vi "dfd_Normalization.vi"(1 "scale type":T1, 2 "h(n)":dbl[](array[numeric])) -> (0 "norm":dbl)   [LabVIEW 2017, in "NI_DigFilterLicensed.lvlib"]
uses:
  <vilib>/addons/Digital Filter Design/NI_DigFilterLicensed.lvlib
  <vilib>/addons/Digital Filter Design/_Objects.llb/DFD Coef Norm Type.ctl
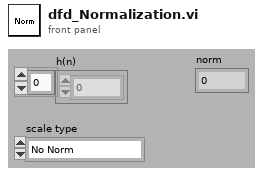
[diagram p1: front panel]
types:
  T1 = typedef "NI_DigFilterLicensed.lvlib/DFD Coef Norm Type.ctl" = enum16{"No Norm", "Time Domain 1-Norm", "Time Domain 2-Norm", "Time Domain Inf-Norm"}
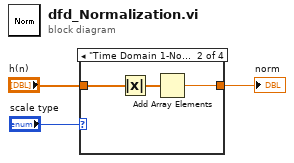
[diagram p0: block diagram]
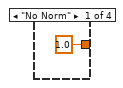
[diagram p2: hidden frame]
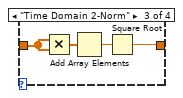
[diagram p3: hidden frame]
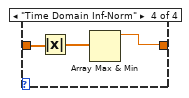
[diagram p4: hidden frame]
diagram:
  n1 = case shown="\"Time Domain 1-Norm\", Default" "scale type" {
    tunnel: "h(n)" -> [_ w7 w11 w14]
    tunnel: [1.0 ("Numeric") w5 w8 w12] -> w3
    frame "No Norm" {
    }
    frame "Time Domain 1-Norm", Default {
      n2 = Absolute Value(x=w7) -> (abs(x)=w6:dbl[])
      n3 = Add Array Elements(numeric array=w6) -> (sum=w5:dbl)
    }
    frame "Time Domain 2-Norm" {
      n4 = Multiply(x=w11, y=w11) -> (x*y=w10:dbl[])
      n5 = Add Array Elements(numeric array=w10) -> (sum=w9:dbl)
      n6 = Square Root(x=w9) -> (sqrt(x)=w8:dbl)
    }
    frame "Time Domain Inf-Norm" {
      n7 = Absolute Value(x=w14) -> (abs(x)=w13:dbl[])
      n8 = Array Max & Min(array=w13) -> (max value=w12:dbl)  [unwired: 3 out]
    }
  }
  "norm" <- w3
